vi "RecordLenghtToRing.vi"(11 "min record length":i32) -> (3 "Record Length (10: 10k points)":u32)   [LabVIEW 2013, in "TektronixDPO.lvclass"]
uses:
  TektronixDPO.lvclass
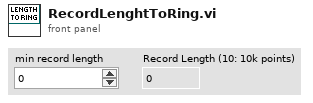
[diagram p1: front panel]
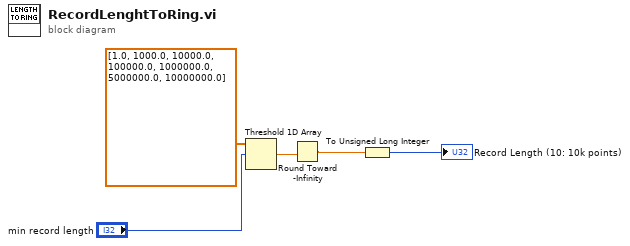
[diagram p0: block diagram]
diagram:
  n1 = Threshold 1D Array(2:"min record length", 3:dbl[] [1.0, 1000.0, 10000.0, 100000.0, 1000000.0, 5000000.0, 10000000.0] ("array of numbers or points")) -> (0:w5:dbl)  [unwired: 1 in]
  n2 = Round Toward -Infinity(1:w5) -> (0:w2:dbl)
  n3 = To Unsigned Long Integer(number=w2) -> (unsigned 32bit integer=→"Record Length (10: 10k points)":u32)
